vi "Read Config.vi"(8 "error in (no error)":errorcluster, 11 "INI":path) -> (0 "error out":errorcluster, 3 "SOL-Config out":refnum<class "SOL-Config.lvclass">)   [LabVIEW 2020, in "Summer of LabVIEW.lvlib" / "SOL-Config.lvclass"]
uses:
  SOL-Config.lvclass
  SOL-Config.lvclass/SOL-Config.ctl
  <vilib>/Utility/config.llb/Read Key (Boolean).vi
  <vilib>/Utility/config.llb/NI_LVConfig.lvlib
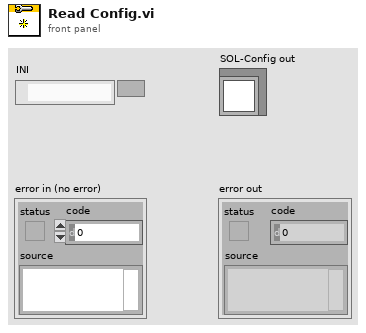
[diagram p1: front panel]
types:
  T1 = typedef "NI_LVConfig.lvlib/Config Data RefNum.ctl" = refnum<k1>
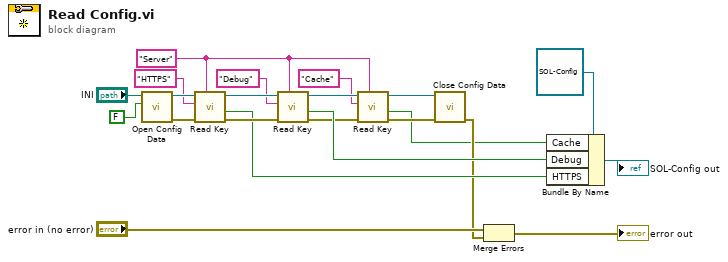
[diagram p0: block diagram]
diagram:
  w4 = "Server" ("section")
  n1 = call <vilib>:"Open Config Data.vi"("create file if necessary (T)"=FALSE, "configuration file path"="INI") -> ("error out"=w19:errorcluster, "refnum"=w20:T1)  [unwired: 7 in, 1 out]
  n2 = call-poly <vilib>:"Read Key.vi"("section"=w4, "error in (no error)"=w19, "key"="HTTPS" ("section"), "refnum"=w20) -> ("error out"=w12:errorcluster, "value"=w10:bool, "refnum out"=w17:T1)  [unwired: 4 in, 1 out]
  n3 = call-poly <vilib>:"Read Key.vi"("section"=w4, "error in (no error)"=w12, "key"="Debug" ("section"), "refnum"=w17) -> ("error out"=w6:errorcluster, "value"=w11:bool, "refnum out"=w7:T1)  [unwired: 4 in, 1 out]
  n4 = call-poly <vilib>:"Read Key.vi"("section"=w4, "error in (no error)"=w6, "key"="Cache" ("section"), "refnum"=w7) -> ("error out"=w2:errorcluster, "value"=w1:bool, "refnum out"=w3:T1)  [unwired: 4 in, 1 out]
  n5 = call <vilib>:"Close Config Data.vi"("error in (no error)"=w2, "refnum"=w3) -> ("error out"=w8:errorcluster)  [unwired: 8 in, 1 out]
  n6 = Merge Errors("error in (no error)", w8) -> (→"error out":errorcluster)
  n7 = Bundle By Name(cluster=refnum<class "SOL-Config.lvclass"> refnum ("SOL-Config in"), "Cache"=w1, "Debug"=w11, "HTTPS"=w10) -> (→"SOL-Config out":refnum<class "SOL-Config.lvclass">)
